vi "2. Module Naming Rules.vi"() -> ()   [LabVIEW 2017]
uses:
  user.lib/_NEVSTOP/Communicable State Machine(CSM)/_Support/Error/CSM Invalid Name Error.vi
  user.lib/_NEVSTOP/Communicable State Machine(CSM)/Communicable State Machine.lvlib
panel:
  in  "Module Name 10":string="parent.module"
  out "error 10":errorcluster={"status"=TRUE, "code"=-1, "source"="\"^module\" is not a valid name."}
  in  "Module Name 9":string=".module"
  out "error 9":errorcluster={"status"=TRUE, "code"=-1, "source"="\"^module\" is not a valid name."}
  out "error 8":errorcluster={"status"=TRUE, "code"=-1, "source"="\"^module\" is not a valid name."}
  in  "Module Name 8":string="^module"
  out "error 7":errorcluster={"status"=TRUE, "code"=-1, "source"="\"^module\" is not a valid name."}
  out "error 6":errorcluster={"status"=TRUE, "code"=-1, "source"="\"module&name\" is not a valid name."}
  out "error 5":errorcluster
  out "error 4":errorcluster
  out "error 3":errorcluster
  out "error 2":errorcluster
  out "error 1":errorcluster
  out "error 0":errorcluster
  in  "Module Name 7":string="^module"
  in  "Module Name 6":string="module&name"
  in  "Module Name 5":string="module-name"
  in  "Module Name 4":string="module_name"
  in  "Module Name 3":string="Module#"
  in  "Module Name 2":string="Group:Module"
  in  "Module Name 1":string="module name"
  in  "Module Name 0":string="Module "
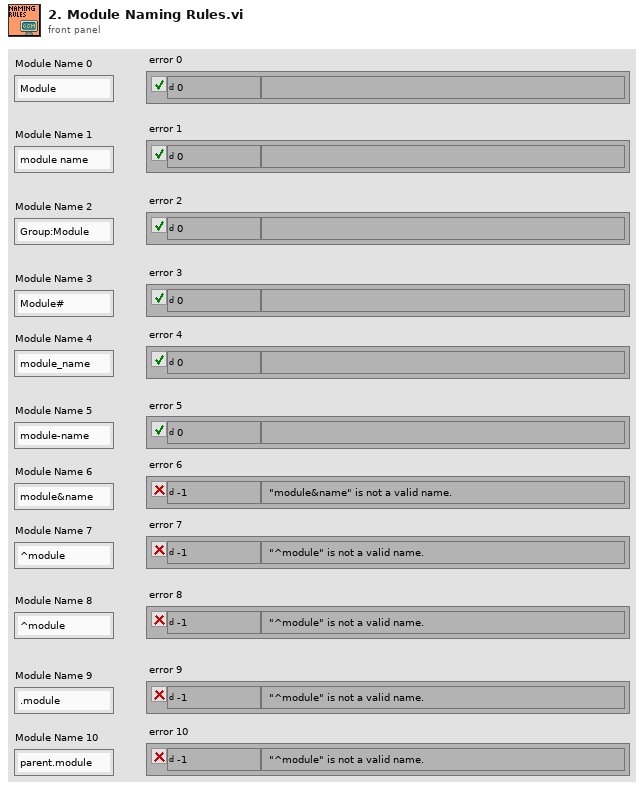
[diagram p1: front panel]
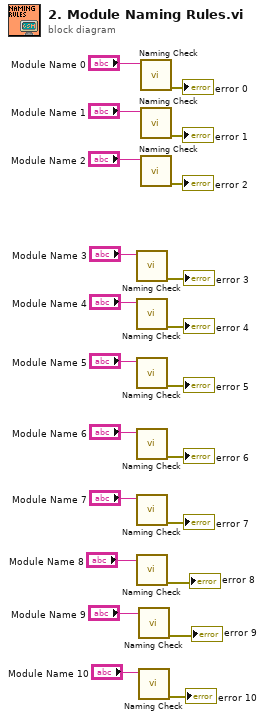
[diagram p0: block diagram]
diagram:
  n1 = call "Naming Check.vi"("Name (\"\" to Use UUID)"="Module Name 3") -> ("error out"=→"error 3":errorcluster)  [unwired: 9 in, 1 out]
  n2 = call "Naming Check.vi"("Name (\"\" to Use UUID)"="Module Name 4") -> ("error out"=→"error 4":errorcluster)  [unwired: 9 in, 1 out]
  n3 = call "Naming Check.vi"("Name (\"\" to Use UUID)"="Module Name 5") -> ("error out"=→"error 5":errorcluster)  [unwired: 9 in, 1 out]
  n4 = call "Naming Check.vi"("Name (\"\" to Use UUID)"="Module Name 6") -> ("error out"=→"error 6":errorcluster)  [unwired: 9 in, 1 out]
  n5 = call "Naming Check.vi"("Name (\"\" to Use UUID)"="Module Name 7") -> ("error out"=→"error 7":errorcluster)  [unwired: 9 in, 1 out]
  n6 = call "Naming Check.vi"("Name (\"\" to Use UUID)"="Module Name 8") -> ("error out"=→"error 8":errorcluster)  [unwired: 9 in, 1 out]
  n7 = call "Naming Check.vi"("Name (\"\" to Use UUID)"="Module Name 9") -> ("error out"=→"error 9":errorcluster)  [unwired: 9 in, 1 out]
  n8 = call "Naming Check.vi"("Name (\"\" to Use UUID)"="Module Name 10") -> ("error out"=→"error 10":errorcluster)  [unwired: 9 in, 1 out]
  n9 = call "Naming Check.vi"("Name (\"\" to Use UUID)"="Module Name 0") -> ("error out"=→"error 0":errorcluster)  [unwired: 9 in, 1 out]
  n10 = call "Naming Check.vi"("Name (\"\" to Use UUID)"="Module Name 1") -> ("error out"=→"error 1":errorcluster)  [unwired: 9 in, 1 out]
  n11 = call "Naming Check.vi"("Name (\"\" to Use UUID)"="Module Name 2") -> ("error out"=→"error 2":errorcluster)  [unwired: 9 in, 1 out]
